vi "sets - add subtract.vi"(10 "array 2":dbl[](array[numeric])=[5.0, 6.0, 7.0, 8.0, 4.0, 5.0, 3.0], 11 "array 1":dbl[](array[numeric])=[1.0, 2.0, 3.0, 4.0]) -> (0 "common array":dbl[](array[numeric])=[4.0], 1 "unified array":dbl[](array[numeric])=[1.0, 2.0, 3.0, 4.0, 5.0, 6.0, 7.0, 8.0])   [LabVIEW 2014]
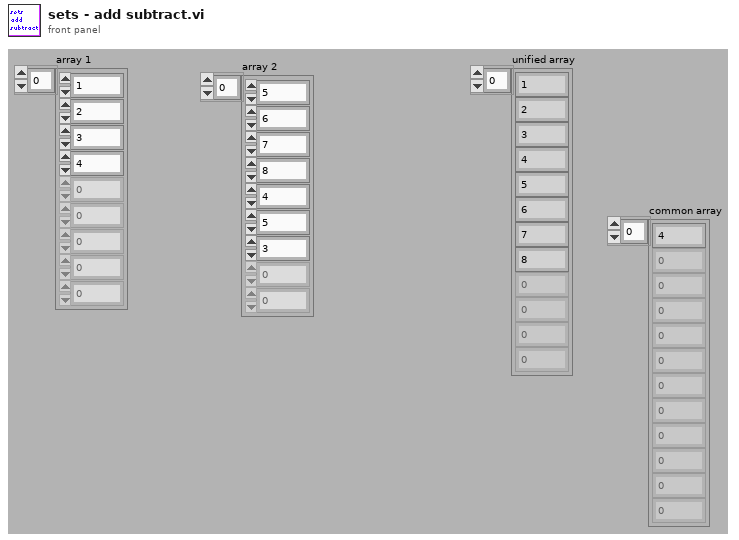
[diagram p1: front panel]
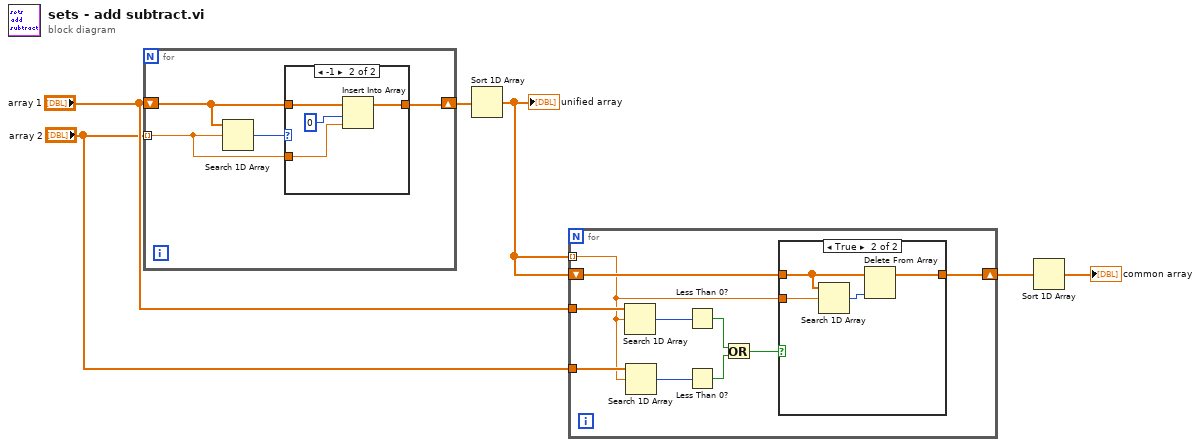
[diagram p0: block diagram]
diagram:
  n1 = for {
    shift-right: [w7] -> w6
    shift-left: "array 1" -> [w9]
    tunnel: "array 2" -> [w8] mode=indexing
    n2 = Search 1D Array(1D array=w9, element=w8) -> (index of element=w10:i32)  [unwired: 1 in]
    n3 = case shown="-1" w10 {
      tunnel: w9 -> [w11 w15]
      tunnel: w8 -> [_ w14]
      tunnel: [w11 w12] -> w7
      frame 0, Default {
      }
      frame -1 {
        n4 = Insert Into Array(array=w15, index=0, new element=w14) -> (w12:dbl[])
      }
    }
  }
  n5 = Sort 1D Array(array=w6) -> (sorted array=w3:dbl[])
  "unified array" <- w3
  n6 = for {
    tunnel: w3 -> [w17] mode=indexing
    shift-right: [w16] -> w1
    shift-left: w3 -> [w18]
    tunnel: "array 1" -> [w25]
    tunnel: "array 2" -> [w24]
    n7 = Search 1D Array(1D array=w25, element=w17) -> (index of element=w23:i32)  [unwired: 1 in]
    n8 = Search 1D Array(1D array=w24, element=w17) -> (index of element=w22:i32)  [unwired: 1 in]
    n9 = Less Than 0?(x=w23) -> (x < 0?=w21:bool)
    n10 = Less Than 0?(x=w22) -> (x < 0?=w20:bool)
    n11 = Or(x=w21, y=w20) -> (x .or. y?=w19:bool)
    n12 = case shown="True" w19 {
      tunnel: w18 -> [w26 w29]
      tunnel: w17 -> [_ w30]
      tunnel: [w26 w27] -> w16
      frame False {
      }
      frame True {
        n13 = Search 1D Array(1D array=w29, element=w30) -> (index of element=w28:i32)  [unwired: 1 in]
        n14 = Delete From Array(array=w29, index=w28) -> (array with subset deleted=w27:dbl[])  [unwired: 1 in, 1 out]
      }
    }
  }
  n15 = Sort 1D Array(array=w1) -> (sorted array=→"common array":dbl[])
